vi "Parse And Set Display Mode.vi"(8 "Error In":errorcluster, 10 "Data":variant, 11 "Display Manager In":refnum<class "Display Manager.lvclass">) -> (0 "Error Out":errorcluster, 3 "Display Manager Out":refnum<class "Display Manager.lvclass">)   [LabVIEW 2019, in "Display Manager.lvclass"]
uses:
  Display Manager.lvclass
  Controls/Display Mode.ctl
  Accessors/Display Mode/Set Display Mode.vi
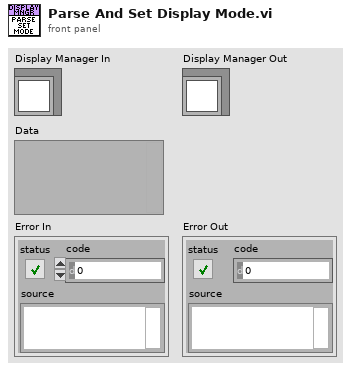
[diagram p1: front panel]
types:
  T1 = typedef "Display Manager.lvclass/Display Mode.ctl" = enum16{"Dashboard", "Audio Analyzer"}
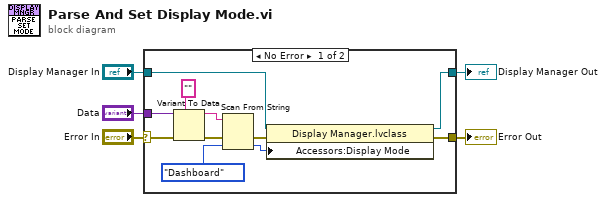
[diagram p0: block diagram]
diagram:
  n1 = case shown="No Error" "Error In" {
    selector: "Error In" -> [w12 w17]
    tunnel: [w16 w17] -> w5
    tunnel: [w15 w18] -> w4
    tunnel: "Display Manager In" -> [w14 w18]
    tunnel: "Data" -> [w13 _]
    frame No Error {
      n2 = Variant To Data(error in=w12, type="", Variant=w13) -> (data=w6:string, error out=w10:errorcluster)
      n3 = Scan From String(input string=w6, error in=w10, default 1=Display_Mode."Dashboard" ("Display Mode")) -> (error out=w7:errorcluster, output 1=w8:T1)  [unwired: 2 in, 2 out]
      n4 = property class="Display Manager.lvclass"(reference=w14, error in=w7, "Accessors:Display Mode"=w8) -> (reference out=w15:refnum<class "Display Manager.lvclass">, error out=w16:errorcluster)
    }
    frame Error {
    }
  }
  "Error Out" <- w5
  "Display Manager Out" <- w4
